vi "Create Test CSV File.vi"() -> ()   [LabVIEW 2015]
uses:
  module/configuration/Sequencer Module configuration.lvclass/Sequencer Module configuration.ctl
  <vilib>/Utility/file.llb/Write Delimited Spreadsheet (string).vi
  classes/Sequence/Config/Sequence Config.lvclass
  Sequencer Module tests.lvlib
  module/configuration/Sequencer Module configuration.lvclass
panel:
  out "Sequence Files Paths":path[](array[path])
  out "error out":errorcluster
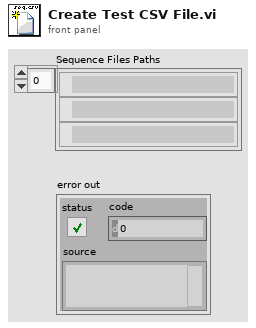
[diagram p1: front panel]
types:
  T1 = typedef "Sequencer Module configuration.lvclass/Line.ctl" = cluster{"Sequence":refnum<class "Sequence Config.lvclass">}
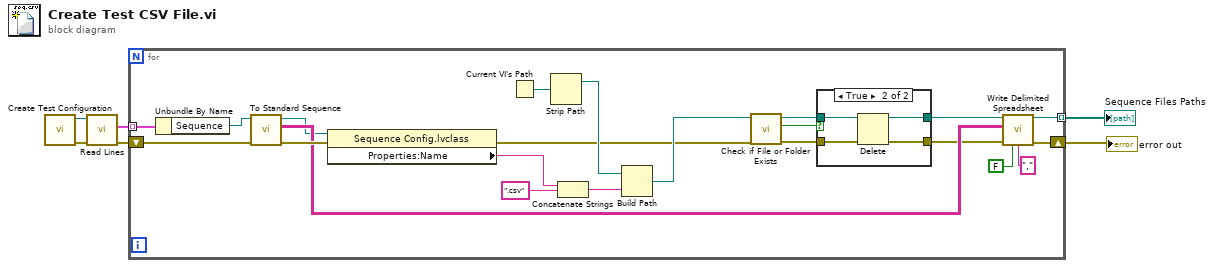
[diagram p0: block diagram]
diagram:
  n1 = call "Create Test Configuration.vi"() -> ("error out"=w4:errorcluster, "Module Configuration"=w5:refnum<class "Sequencer Module configuration.lvclass">)  [unwired: 6 in, 4 out]
  n2 = call "Read Lines.vi"("error in (no error)"=w4, "Sequencer Module configuration in"=w5) -> ("error out"=w3:errorcluster, "Lines"=w6:T1[])  [unwired: 7 in, 1 out]
  n3 = for {
    tunnel: w6 -> [w28] mode=indexing
    shift-right: [w26] -> w2
    shift-left: w3 -> [w27]
    tunnel: [w21] -> w1 mode=indexing
    n4 = Unbundle By Name(w28) -> ("Sequence"=w25:refnum<class "Sequence Config.lvclass">)
    n5 = call-dynamic "To Standard Sequence.vi"("error in (no error)"=w27, "Sequence Config in"=w25) -> ("error out"=w22:errorcluster, "Standard Sequence"=w16:string[][], "Sequence Config out"=w14:refnum<class "Sequence Config.lvclass">)  [unwired: 7 in]
    n6 = property class="Sequence Config.lvclass"(reference=w14, error in=w22) -> (error out=w10:errorcluster, "Properties:Name"=w19:string)  [unwired: 1 out]
    n7 = Current VI's Path() -> (path=w24:path)
    n8 = Strip Path(path=w24) -> (stripped path=w23:path)  [unwired: 1 out]
    n9 = Concatenate Strings(w19, ".csv" ("string")) -> (w18:string)
    n10 = Build Path(base path=w23, name or relative path=w18) -> (appended path=w13:path)
    n11 = call <vilib>:"Check if File or Folder Exists.vi"("error in (no error)"=w10, "path"=w13) -> ("error out"=w8:errorcluster, "file or folder exists?"=w12:bool, "dup path"=w11:path)  [unwired: 7 in]
    n12 = case shown="True" w12 {
      tunnel: w11 -> [w30 w34]
      tunnel: [w30 w33] -> w9
      tunnel: w8 -> [w29 w32]
      tunnel: [w29 w31] -> w7
      frame False {
      }
      frame True {
        n13 = Delete(path (use dialog)=w34, error in=w32) -> (deleted path=w33:path, error out=w31:errorcluster)  [unwired: 3 in, 1 out]
      }
    }
    n14 = call-poly <vilib>:"Write Delimited Spreadsheet.vi"("file path (dialog if empty)"=w9, "2D data"=w16, "error in (no error)"=w7, "transpose? (F)"=FALSE, "delimiter (\\t)"="," ("delimiter (\\t)")) -> ("new file path (Not A Path if cancelled)"=w21:path, "error out"=w26:errorcluster)  [unwired: 9 in]
  }
  "error out" <- w2
  "Sequence Files Paths" <- w1
